vi "WPI_SolenoidOpen.vi"   [LabVIEW 2017]
doc: "Opens a reference to the solenoid you specify. You must open a reference before using any other VIs on this palette.\n\nSelect \"Single\" if your solenoid has 1 coil. Select \"Double\" if your solenoid has 2 coils.\n\nThis software is licensed. Open the labview\\readme\\WPI Robotics Library Open Source License.txt file for more information."
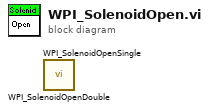
[diagram p0: block diagram]
diagram:
  n1 = call <vilib>:"WPI_SolenoidOpenDouble.vi"() -> ()  [unwired: 10 in, 2 out]
  n2 = call <vilib>:"WPI_SolenoidOpenSingle.vi"() -> ()  [unwired: 10 in, 2 out]
